vi "AutoTurn.vi"(8 "error in (no error)":errorcluster, 9 "TimeOut (s)":dbl, 10 "MaxSpeed (ft/s)":dbl, 11 "degrees":dbl) -> (0 "error out":errorcluster)   [LabVIEW 2020]
doc: "Turn for auto\ninputs:\n--Timer\n-error in\n\noutputs:\n--error out"
uses:
  <vilib>/Utility/semaphor.llb/Obtain Semaphore Reference.vi
  <vilib>/Rock Robotics/WPI/ThirdParty/JAS_Junk/TrajLib/Timer_Reset.vi
  <vilib>/Rock Robotics/WPI/ThirdParty/JAS_Junk/TrajLib/Trajectory_Library.lvlib
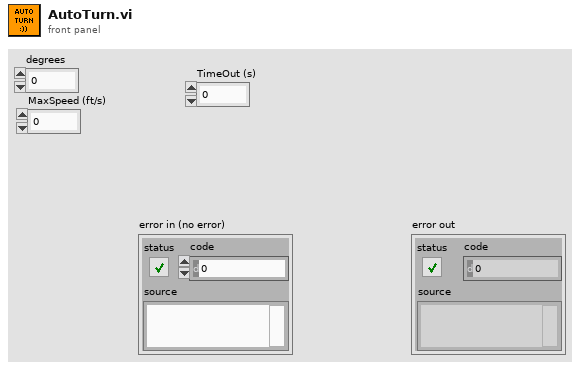
[diagram p1: front panel]
types:
  T1 = typedef "Trajectory_Library.lvlib/TIMER.ctl" = cluster{"StartTime":dbl, "Accumulated TIme":dbl, "Running":bool, "semaphore":T2}
  T2 = typedef "Semaphore RefNum" = refnum<k1>
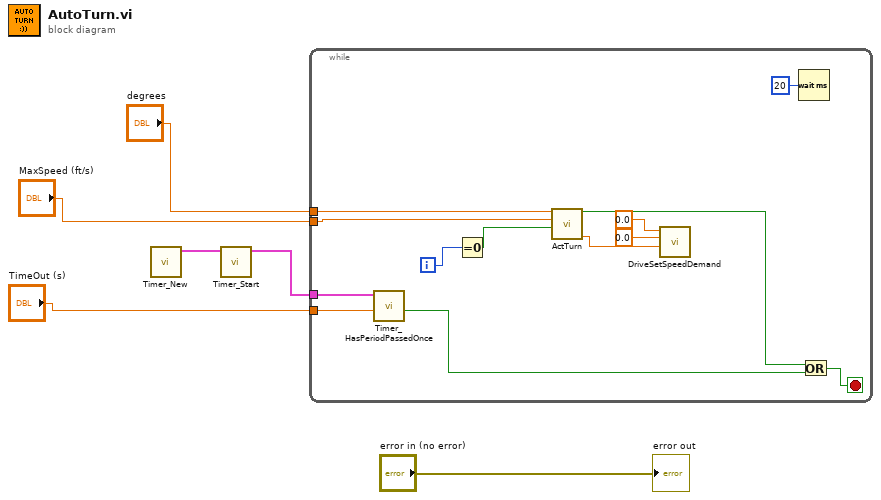
[diagram p0: block diagram]
diagram:
  n1 = call <vilib>:"Timer_New.vi"() -> ("TIMER"=w3:T1)  [unwired: 11 in]
  n2 = call <vilib>:"Timer_Start.vi"("in Timer"=w3) -> ("out Timer"=w2:T1)  [unwired: 10 in]
  n3 = while {
    tunnel: "degrees" -> [w13]
    tunnel: "MaxSpeed (ft/s)" -> [w12]
    tunnel: w2 -> [w18]
    tunnel: "TimeOut (s)" -> [w17]
    i -> [w19]
    stop <- w15 stop-if-true
    n4 = call <vilib>:"Timer_HasPeriodPassedOnce.vi"("Period"=w17, "in Timer"=w18) -> ("Expired"=w16:bool)  [unwired: 7 in, 2 out]
    n5 = Equal To 0?(x=w19) -> (x = 0?=w11:bool)
    n6 = call "ActTurn.vi"("FirstTime"=w11, "MaxSpeed (ft/s)"=w12, "Degrees"=w13) -> ("RightSpeedDemand"=w9:dbl, "Done"=w10:bool)  [unwired: 6 in, 1 out]
    n7 = call "DriveSetSpeedDemand.vi"("ASpeedDemand (d/s)"=w9, "YSpeedDemand (ft/s)"=0.0, "XSpeedDemand (ft/s)"=0.0) -> ()  [unwired: 9 in]
    n8 = Wait (ms)(milliseconds to wait=u32 20) -> ()  [unwired: 1 out]
    n9 = Or(x=w10, y=w16) -> (x .or. y?=w15:bool)
  }
  "error out" <- "error in (no error)"
